vi "AlliGator Compute Decay Statistics v2.vi"(7 "Decay Statistics Bin":i32=1 min=1, 8 "Error In":errorcluster, 9 "Current Data":refnum<vi>, 10 "Image Array":T1[](array[typedef]), 11 "Decay Statistics Graph Ref":refnum<vi>) -> (0 "Error Out":errorcluster, 1 "Message":string, 2 "Decays Min Values":sgl[](array[numeric]), 3 "Decays Max Values":sgl[](array[numeric]), 4 "Time (s)":dbl)   [LabVIEW 2021, in "AlliGator Decay Statistics.lvlib"]
doc: "Computes decay min & max histograms."
uses:
  AlliGator Decay Statistics.lvlib
  <vilib>/vision/Image Controls.llb/IMAQ Image.ctl
  Histograms/Linear Histogram Options.ctl
  Histograms/Histogram Bin Option.ctl
  Histograms/Histogram Bin Position.ctl
  33da87fb-858f-4a51-b06a-087e09af93f3.vi
  cb8872dc-784b-405f-8a79-31bbf4f66ef6.vi
  33da87fb-858f-4a51-b06a-087e09af93f3.vi/e021cd17-e000-4244-b7f4-ec50548bdfcb.vi
  33da87fb-858f-4a51-b06a-087e09af93f3.vi/b1828c6e-eb0a-43e9-a724-8b596c52e435.vi
  33da87fb-858f-4a51-b06a-087e09af93f3.vi/7a6138ed-c001-4311-b538-9ba42ae7c7b1.vi
  33da87fb-858f-4a51-b06a-087e09af93f3.vi/52c6b4fa-501b-4af0-803b-8bab516ca5d3.vi
  33da87fb-858f-4a51-b06a-087e09af93f3.vi/d7237e10-35ab-4bcb-a0c6-4883c3f4c990.vi
  33da87fb-858f-4a51-b06a-087e09af93f3.vi/5fb5dd96-3b97-4592-ba56-58181c8e7105.vi
  33da87fb-858f-4a51-b06a-087e09af93f3.vi/8e13a849-a393-4484-9968-4af7b25c38d7.vi
  cb8872dc-784b-405f-8a79-31bbf4f66ef6.vi/e021cd17-e000-4244-b7f4-ec50548bdfcb.vi
  cb8872dc-784b-405f-8a79-31bbf4f66ef6.vi/b1828c6e-eb0a-43e9-a724-8b596c52e435.vi
  cb8872dc-784b-405f-8a79-31bbf4f66ef6.vi/7a6138ed-c001-4311-b538-9ba42ae7c7b1.vi
  cb8872dc-784b-405f-8a79-31bbf4f66ef6.vi/52c6b4fa-501b-4af0-803b-8bab516ca5d3.vi
  cb8872dc-784b-405f-8a79-31bbf4f66ef6.vi/d7237e10-35ab-4bcb-a0c6-4883c3f4c990.vi
  cb8872dc-784b-405f-8a79-31bbf4f66ef6.vi/5fb5dd96-3b97-4592-ba56-58181c8e7105.vi
  cb8872dc-784b-405f-8a79-31bbf4f66ef6.vi/8e13a849-a393-4484-9968-4af7b25c38d7.vi
  Globals, Variables, Constants/AlliGator Abort.vi
  <vilib>/vision/EDVR.llb/IMAQ ImageToEDVR 2D U8.vi
  <vilib>/vision/EDVR.llb/IMAQ ImageToEDVR 2D I16.vi
  <vilib>/vision/EDVR.llb/IMAQ ImageToEDVR 2D SGL.vi
  <vilib>/vision/EDVR.llb/IMAQ ImageToEDVR 2D U16.vi
  <userlib>/_OpenG.lib/array/array.llb/Filter 1D Array__ogtk.vi
  <userlib>/_OpenG.lib/array/array.llb/Filter 1D Array (DBL)__ogtk.vi
  <userlib>/_OpenG.lib/array/array.llb/Delete Elements from Array__ogtk.vi
  <userlib>/_OpenG.lib/array/array.llb/Delete Elements from 1D Array (DBL)__ogtk.vi
  <vilib>/Utility/error.llb/Error Cluster From Error Code.vi
  Graphs/XY Graph/XY Graph Add Single Plot with Name.vi
  <vilib>/ErrorRing/Error Ring.xnode
  Graphs/XY Graph/XY Graph Add-Ons.lvlib
  Time/Time.lvlib
  Globals, Variables, Constants/AlliGator Globals, Variables & Constants.lvlib
  Histograms/Histogram Window.lvlib
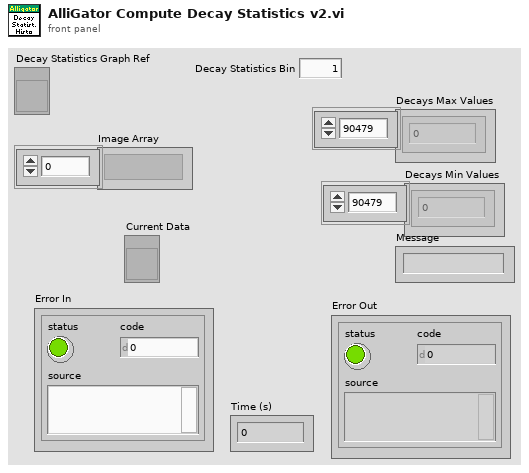
[diagram p1: front panel]
types:
  T1 = typedef "IMAQ Image.ctl" = refnum<image>
  T2 = typedef "Histogram Window.lvlib/Linear Histogram Options.ctl" = cluster{"Bin Size":dbl, "Bin Number":i32, "Bin Option":T3, "Min Value":dbl, "Max Value":dbl, "Filter NaN & Infinite Values":bool, "Frequency Plot":bool, "Align Bins":bool, "Bin Location":T4, "Project Outside Values":bool, "Max Histogram Size":i32}
  T3 = typedef "Histogram Window.lvlib/Histogram Bin Option.ctl" = enum32{"Bin Number", "Bin Size"}
  T4 = typedef "Histogram Window.lvlib/Histogram Bin Position.ctl" = enum16{"Left", "Center", "Right"}
  T5 = typedef "Image Type" = u32
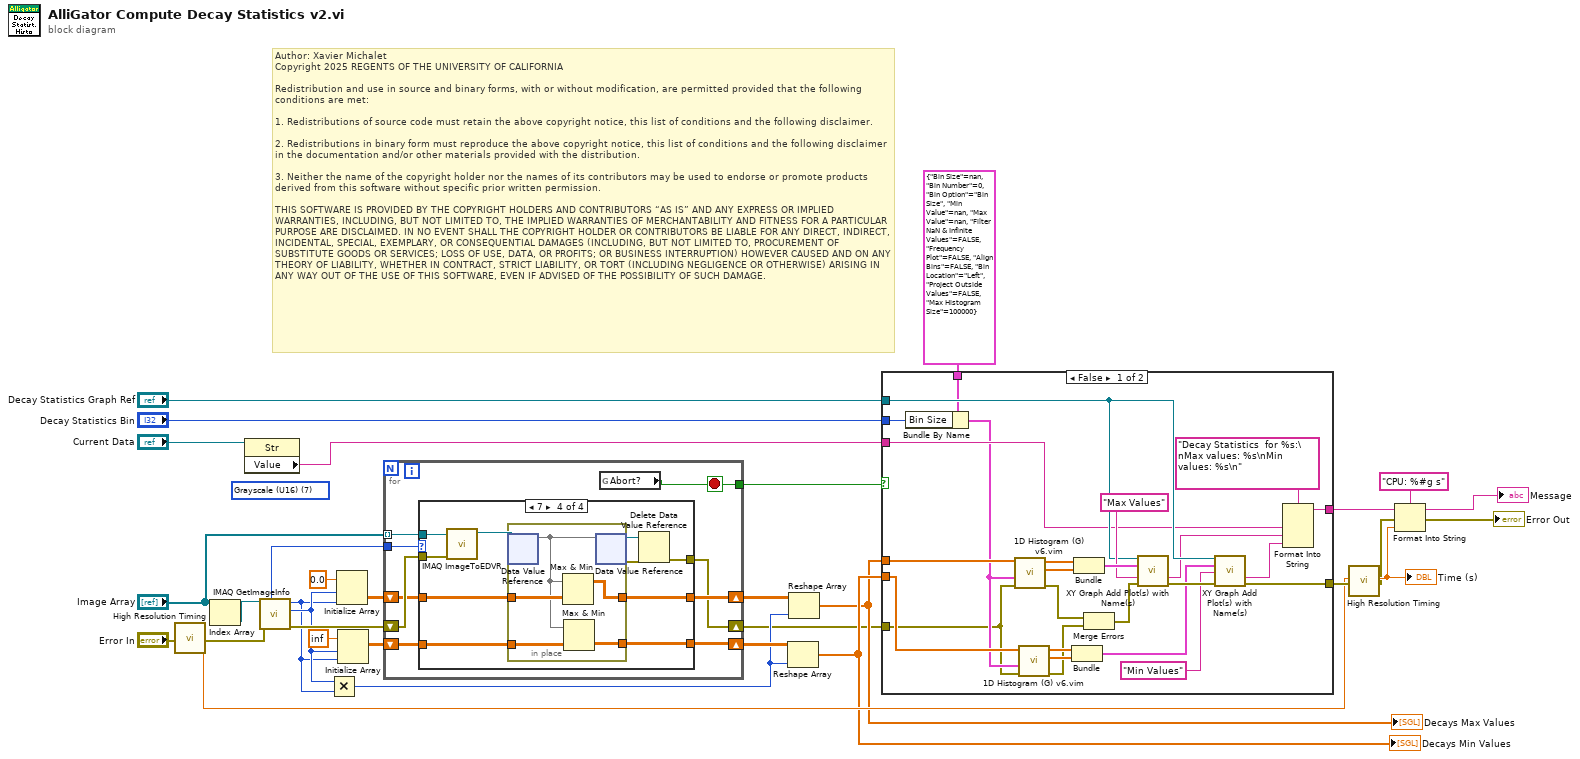
[diagram p0: block diagram]
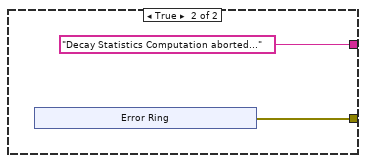
[diagram p2: hidden frame]
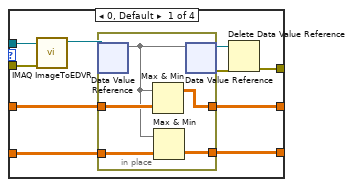
[diagram p3: hidden frame]
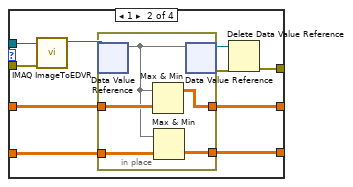
[diagram p4: hidden frame]
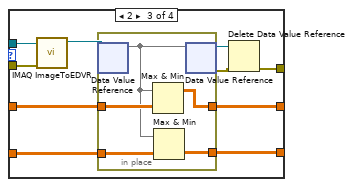
[diagram p5: hidden frame]
diagram:
  (unwired) T5 7 items=["Grayscale (U8)", "Grayscale (I16)", "Grayscale (SGL)", "Complex (CSG)", "RGB (U32)", "HSL (U32)", "RGB (U64)", "Grayscale (U16)"] ("Image Type")
  # "Author: Xavier Michalet\nCopyright 2025 REGENTS OF THE UNIVERSITY OF CALIFORNIA\n\nRedistribution and use in source and binary forms, with or without modification, are permitted provided that the following conditions are met:\n\n1. Redistributions of source code must retain the above copyright notice, this list of conditions and the following disclaimer.\n\n2. Redistributions in binary form must reproduce the above copyright notice, this list of conditions and the following disclaimer in the documentation and/or other materials provided with the distribution.\n\n3. Neither the name of the copyright holder nor the names of its contributors may be used to endorse or promote products derived from this software without specific prior written permission.\n\nTHIS SOFTWARE IS PROVIDED BY THE COPYRIGHT HOLDERS AND CONTRIBUTORS “AS IS” AND ANY EXPRESS OR IMPLIED WARRANTIES, INCLUDING, BUT NOT LIMITED TO, THE IMPLIED WARRANTIES OF MERCHANTABILITY AND FITNESS FOR A PARTICULAR PURPOSE ARE DISCLAIMED. IN NO EVENT SHALL THE COPYRIGHT HOLDER OR CONTRIBUTORS BE LIABLE FOR ANY DIRECT, INDIRECT, INCIDENTAL, SPECIAL, EXEMPLARY, OR CONSEQUENTIAL DAMAGES (INCLUDING, BUT NOT LIMITED TO, PROCUREMENT OF SUBSTITUTE GOODS OR SERVICES; LOSS OF USE, DATA, OR PROFITS; OR BUSINESS INTERRUPTION) HOWEVER CAUSED AND ON ANY THEORY OF LIABILITY, WHETHER IN CONTRACT, STRICT LIABILITY, OR TORT (INCLUDING NEGLIGENCE OR OTHERWISE) ARISING IN ANY WAY OUT OF THE USE OF THIS SOFTWARE, EVEN IF ADVISED OF THE POSSIBILITY OF SUCH DAMAGE."
  n1 = call "High Resolution Timing.vi"("Error In"="Error In") -> ("elapsed (relative) seconds"=w22:dbl, "Error Out"=w24:errorcluster)  [unwired: 16 in, 1 out]
  n2 = Index Array(array="Image Array") -> (element=w31:T1)  [unwired: 1 in]
  n3 = property class="Str"(reference="Current Data") -> ("Value"=w5:string)  [unwired: 1 in, 2 out]
  n4 = call "IMAQ GetImageInfo"("error in (no error)"=w24, "Image"=w31) -> ("error out"=w29:errorcluster, "Y Resolution"=w7:i32, "X Resolution"=w6:i32, "Image Type"=w11:T5)  [unwired: 2 in, 4 out]
  n5 = Multiply(x=w7, y=w6) -> (x*y=w14:i32)
  n6 = Initialize Array(0.0 ("element"), w7, w6) -> (w17:dbl[][])
  n7 = Initialize Array(inf ("element"), w7, w6) -> (w9:dbl[][])
  n8 = for {
    tunnel: "Image Array" -> [w41] mode=indexing
    tunnel: [w33] -> w25
    shift-right: [w37] -> w15
    shift-left: w17 -> [w38]
    shift-right: [w35] -> w16
    shift-left: w9 -> [w36]
    tunnel: w11 -> [w40]
    shift-right: [w34] -> w10
    shift-left: w29 -> [w39]
    stop <- w33 stop-if-true
    n9 = case shown="7" w40 {
      tunnel: w41 -> [w51 w66 w81 w96]
      tunnel: w39 -> [w50 w65 w80 w95]
      tunnel: w38 -> [w47 w62 w77 w92]
      tunnel: [w46 w61 w76 w91] -> w37
      tunnel: w36 -> [w45 w60 w75 w90]
      tunnel: [w44 w59 w74 w89] -> w35
      tunnel: [w42 w57 w72 w87] -> w34
      frame 0, Default {
        n10 = call-poly <vilib>:"IMAQ ImageToEDVR.vi"("error in (no error)"=w50, "Image"=w51) -> ("EDVR 2D U8"=w49:refnum<data-value>)  [unwired: 7 in, 2 out]
        n11 = in-place {
          in-place-border: w47 -> [w56]
          in-place-border: [w55] -> w46
          in-place-border: w45 -> [w54]
          in-place-border: [w53] -> w44
          n12 = in-place-dvr #1(w49) -> (w52:u8[][])  [unwired: 1 out]
          n13 = Max & Min(x=w52, y=w56) -> (max(x,y)=w55:dbl[][])  [unwired: 1 out]
          n14 = Max & Min(x=w52, y=w54) -> (min(x,y)=w53:dbl[][])  [unwired: 1 out]
          n15 = in-place-dvr #1(w52) -> (w48:refnum<data-value>, w43:errorcluster)
        }
        n16 = Delete Data Value Reference(data value reference=w48, error in=w43) -> (error out=w42:errorcluster)  [unwired: 1 out]
      }
      frame 1 {
        n17 = call-poly <vilib>:"IMAQ ImageToEDVR.vi"("error in (no error)"=w65, "Image"=w66) -> ("EDVR 2D I16"=w64:refnum<data-value>)  [unwired: 7 in, 2 out]
        n18 = in-place {
          in-place-border: w62 -> [w71]
          in-place-border: [w70] -> w61
          in-place-border: w60 -> [w69]
          in-place-border: [w68] -> w59
          n19 = in-place-dvr #2(w64) -> (w67:i16[][])  [unwired: 1 out]
          n20 = Max & Min(x=w67, y=w71) -> (max(x,y)=w70:dbl[][])  [unwired: 1 out]
          n21 = Max & Min(x=w67, y=w69) -> (min(x,y)=w68:dbl[][])  [unwired: 1 out]
          n22 = in-place-dvr #2(w67) -> (w63:refnum<data-value>, w58:errorcluster)
        }
        n23 = Delete Data Value Reference(data value reference=w63, error in=w58) -> (error out=w57:errorcluster)  [unwired: 1 out]
      }
      frame 2 {
        n24 = call-poly <vilib>:"IMAQ ImageToEDVR.vi"("error in (no error)"=w80, "Image"=w81) -> ("EDVR 2D SGL"=w79:refnum<data-value>)  [unwired: 7 in, 2 out]
        n25 = in-place {
          in-place-border: w77 -> [w86]
          in-place-border: [w85] -> w76
          in-place-border: w75 -> [w84]
          in-place-border: [w83] -> w74
          n26 = in-place-dvr #3(w79) -> (w82:sgl[][])  [unwired: 1 out]
          n27 = Max & Min(x=w82, y=w86) -> (max(x,y)=w85:dbl[][])  [unwired: 1 out]
          n28 = Max & Min(x=w82, y=w84) -> (min(x,y)=w83:dbl[][])  [unwired: 1 out]
          n29 = in-place-dvr #3(w82) -> (w78:refnum<data-value>, w73:errorcluster)
        }
        n30 = Delete Data Value Reference(data value reference=w78, error in=w73) -> (error out=w72:errorcluster)  [unwired: 1 out]
      }
      frame 7 {
        n31 = call-poly <vilib>:"IMAQ ImageToEDVR.vi"("error out"=w95, "Image"=w96) -> ("EDVR 2D U16"=w94:refnum<data-value>)  [unwired: 7 in, 2 out]
        n32 = in-place {
          in-place-border: w92 -> [w101]
          in-place-border: [w100] -> w91
          in-place-border: w90 -> [w99]
          in-place-border: [w98] -> w89
          n33 = in-place-dvr #4(w94) -> (w97:u16[][])  [unwired: 1 out]
          n34 = Max & Min(x=w97, y=w101) -> (max(x,y)=w100:dbl[][])  [unwired: 1 out]
          n35 = Max & Min(x=w97, y=w99) -> (min(x,y)=w98:dbl[][])  [unwired: 1 out]
          n36 = in-place-dvr #4(w97) -> (w93:refnum<data-value>, w88:errorcluster)
        }
        n37 = Delete Data Value Reference(data value reference=w93, error in=w88) -> (error out=w87:errorcluster)  [unwired: 1 out]
      }
    }
    n38 = global read "AlliGator Abort.vi" "Abort?"() -> (w33:bool)
  }
  n39 = Reshape Array(w16, w14) -> (w13:dbl[])
  "Decays Min Values" <- w13
  n40 = Reshape Array(w15, w14) -> (w12:dbl[])
  "Decays Max Values" <- w12
  n41 = case shown="False" w25 {
    tunnel: w12 -> [w126 _]
    tunnel: w13 -> [w120 _]
    tunnel: "Decay Statistics Bin" -> [w108 _]
    tunnel: "Decay Statistics Graph Ref" -> [w116 _]
    tunnel: [w115 w128] -> w26
    tunnel: [w113 "Decay Statistics Computation aborted..."] -> w21
    tunnel: w5 -> [w111 _]
    tunnel: w10 -> [w105 _]
    tunnel: T2 {"Bin Size"=nan, "Bin Number"=0, "Bin Option"=enum."Bin Size", "Min Value"=nan, "Max Value"=nan, "Filter NaN & Infinite Values"=FALSE, "Frequency Plot"=FALSE, "Align Bins"=FALSE, "Bin Location"=enum."Left", "Project Outside Values"=FALSE, "Max Histogram Size"=100000} ("Histogram Options") -> [w107 _]
    frame False {
      n42 = Bundle By Name(cluster=w107, "Bin Size"=w108) -> (w106:T2)
      n43 = call "1D Histogram (G) v6.vim"("Error In"=w105, "Histogram Options"=w106, "Array"=w126) -> ("Error Out"=w102:errorcluster, "Histogram"=w124:dbl[], "Axis"=w125:dbl[])  [unwired: 2 in, 4 out]
      n44 = call "1D Histogram (G) v6.vim"("Error In"=w105, "Histogram Options"=w106, "Array"=w120) -> ("Error Out"=w103:errorcluster, "Histogram"=w118:dbl[], "Axis"=w119:dbl[])  [unwired: 2 in, 4 out]
      n45 = Bundle("Axis"=w119, "Histogram"=w118) -> (w117:cluster{"Axis":dbl[], "Histogram":dbl[]})  [unwired: 1 in]
      n46 = Bundle("Axis"=w125, "Histogram"=w124) -> (w123:cluster{"Axis":dbl[], "Histogram":dbl[]})  [unwired: 1 in]
      n47 = Merge Errors(w102, w103) -> (w104:errorcluster)
      n48 = call-poly "XY Graph Add Plot(s) with Name(s).vi"("XYGraph Ref in"=w116, "Plot"=w123, "Plot Name (\"Plot\")"="Max Values" ("Plot Name (\"Plot\")"), "error in (no error)"=w104) -> ("Plot Name"=w110:string, "error out"=w121:errorcluster)  [unwired: 8 in, 2 out]
      n49 = call-poly "XY Graph Add Plot(s) with Name(s).vi"("XYGraph Ref in"=w116, "Plot"=w117, "Plot Name (\"Plot\")"="Min Values" ("Plot Name (\"Plot\")"), "error in (no error)"=w121) -> ("Plot Name"=w109:string, "error out"=w115:errorcluster)  [unwired: 8 in, 2 out]
      n50 = Format Into String(format string="Decay Statistics  for %s:\nMax values: %s\nMin values: %s\n", w111, w110, w109) -> (resulting string=w113:string)  [unwired: 2 in, 1 out]
    }
    frame True {
      n51 = xnode "Error Ring"() -> ("error out"=w128:errorcluster)
    }
  }
  n52 = call "High Resolution Timing.vi"("relative seconds (NaN)"=w22, "Error In"=w26) -> ("elapsed (relative) seconds"=w20:dbl, "Error Out"=w3:errorcluster)  [unwired: 15 in, 1 out]
  "Time (s)" <- w20
  n53 = Format Into String(format string="CPU: %#g s", initial string=w21, error in=w3, w20) -> (resulting string=→"Message":string, error out=→"Error Out":errorcluster)
